vi "wrapandcutmultimages.vi"(0 "rasterscanned array":sgl[](array[numeric])) -> (1 "imagearray":sgl[][](array[numeric]), 2 "wrap":i32)   [LabVIEW 2013]
panel:
  out "appended array":dbl[][](array[numeric])
  in  "Array":dbl[][](array[numeric])
  out "P":dbl
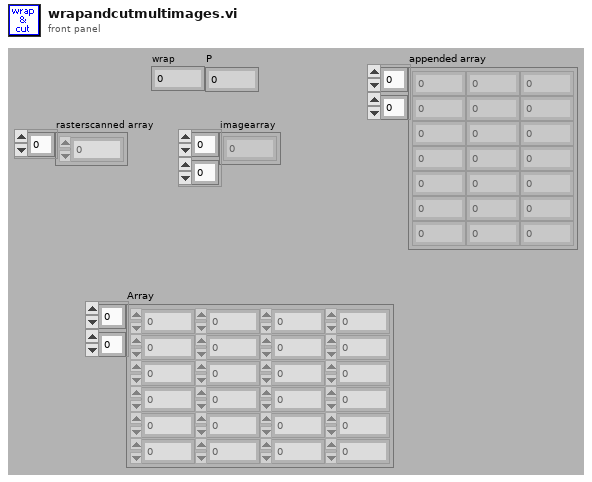
[diagram p1: front panel]
types:
  T1 = typedef "LVRectTypeDef.ctl" = cluster{"Left":i16, "Top":i16, "Right":i16, "Bottom":i16}
  T2 = cluster{"Xpixels":i32, "Vxminref":dbl, "Vxmaxref":dbl, "P":dbl, "Ypixels":i32, "Vyminref":dbl, "Vymaxref":dbl, "srate":sgl, "sAOxy":i32, "timeout":dbl, "type":string, "date":string, "time":string, "Colormap":u16, "Drawing Mode":u16, "Scanning Mode":u16, "square pixels":bool, "square matrix":bool, "Xpixels Img":i32, "Vx-min Img":dbl, "VX-max Img":dbl, "Ypixels Img":i32, "Vy-min Img":dbl, "Vy-max Img ":dbl, "Angle Img":dbl, "autoshutter":bool, "finite":bool, "cont":bool, "wavdet":bool, "measpoints":i32, "avpp":i32, "bufferAO":i32, "bufferAI":i32, "starttick":u32, "waveform":path, "Vx-ref":dbl, "Vy-ref":dbl, "refreshrate":dbl, "refreshbuffer":i32, "tt_cycles":i32, "motorref":refnum<k7>, "mirrorswitch":refnum<k7>, "sample mode":i32, "maxbufferAI":i32, "sampletreshold":dbl, "srateAODO":sgl, "bin":sgl, "Pel":sgl, "Angle draw":dbl, "srate Img":sgl, "ROIimg_plotbounds":T1, "auto OD":bool, "ODfilt":u16, "reset AO_DO":bool, "aAI":i32[], "aCI":i32[], "aAO":i32[], "aDO":i32[]}
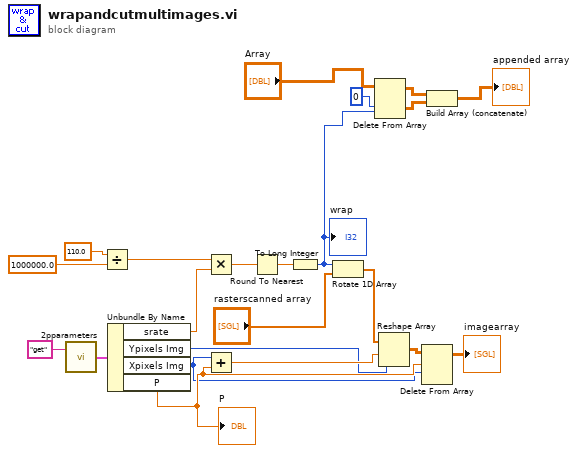
[diagram p0: block diagram]
diagram:
  n1 = call "2pparameters.vi"("command"="get") -> ("params out"=w21:T2)  [unwired: 1 in]
  n2 = Divide(x=110.0, y=1000000.0) -> (x/y=w15:dbl)
  n3 = Unbundle By Name(w21) -> ("srate"=w14:sgl, "Ypixels Img"=w8:i32, "Xpixels Img"=w7:i32, "P"=w22:dbl)
  "P" <- w22
  n4 = Multiply(x=w15, y=w14) -> (x*y=w10:dbl)
  n5 = Add(x=w7, y=w22) -> (x+y=w9:dbl)
  n6 = Round To Nearest(number=w10) -> (nearest integer value=w13:dbl)
  n7 = To Long Integer(number=w13) -> (32bit integer=w1:i32)
  "wrap" <- w1
  n8 = Rotate 1D Array(1:"rasterscanned array", 2:w1) -> (0:w11:sgl[])
  n9 = Delete From Array(array="Array", length=w1, index (row)=0 ("index")) -> (deleted portion=w5:dbl[][], array with subset deleted=w3:dbl[][])  [unwired: 1 in]
  n10 = Reshape Array(w11, w9, w8) -> (w18:sgl[][])
  n11 = Delete From Array(array=w18, length=w22, index (row)=w7) -> (array with subset deleted=→"imagearray":sgl[][])  [unwired: 1 in, 1 out]
  n12 = Build Array (concatenate)(w3, w5) -> (→"appended array":dbl[][])
